vi "_f_IEEE754formatReverse.vi"(8 "error in (no error)":errorcluster, 9 "Number":sgl=-101.101 format="%.2f") -> (0 "error out":errorcluster, 1 "String":string="459CFFAE")   [LabVIEW 2013]
doc: "This VI shows how LabVIEW stores SGL floating-point numbers in memory in binary format. The 32-bit binary number is based on the following IEEE 754 format:\n\n1 bit for the SIGN\n8 bits for the EXPONENT\n23 bits for the MANTISSA\n\nThe formula for the conversion is the following:\n\nSGL = (-1)^SIGN * 1.MANTISSA * 2^(EXPONENT-127)\n\nYou can use this VI to convert SGL numbers to their binary storage equivalent, and vice versa."
panel:
  # "SGL to Binary Storage Format"
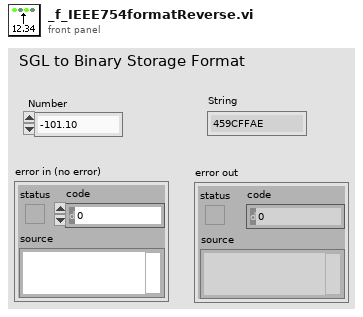
[diagram p1: front panel]
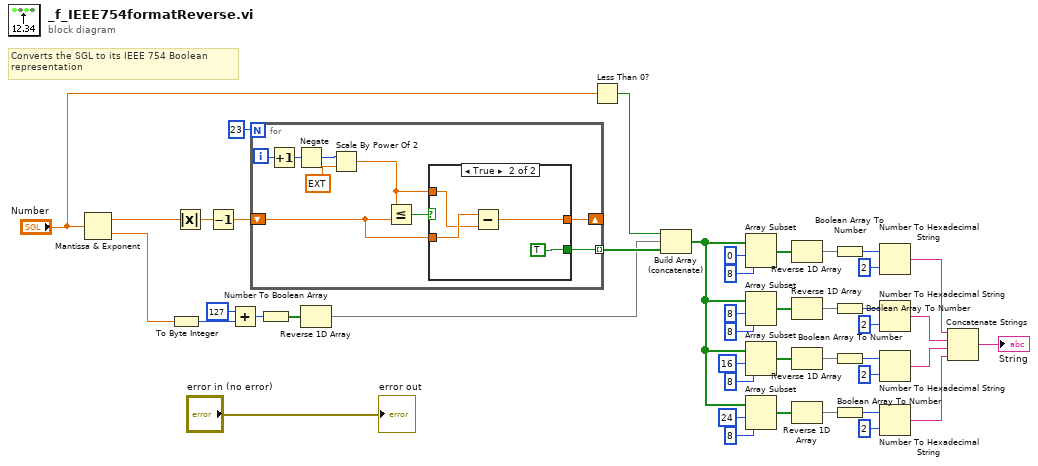
[diagram p0: block diagram]
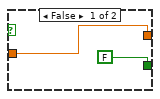
[diagram p2: hidden frame]
diagram:
  # "Converts the SGL to its IEEE 754 Boolean \nrepresentation"
  n1 = Mantissa & Exponent(0:"Number") -> (1:w35:sgl, 2:w38:sgl)
  n2 = To Byte Integer(number=w38) -> (8bit integer=w44:i8)
  n3 = Absolute Value(x=w35) -> (abs(x)=w36:sgl)
  n4 = Decrement(x=w36) -> (x-1=w40:sgl)
  n5 = Add(x=i8 127, y=w44) -> (x+y=w43:i8)
  n6 = for {
    N: 23 -> [_]
    shift-right: [w46] -> _
    shift-left: w40 -> [w48]
    tunnel: [w45] -> w33 mode=indexing
    i -> [w53]
    n7 = Increment(x=w53) -> (x+1=w52:i32)
    n8 = Negate(x=w52) -> (-x=w51:i32)
    n9 = Scale By Power Of 2(n=w51, x=ext 1.0) -> (x*2^n=w47:ext)
    n10 = Less Or Equal?(x=w47, y=w48) -> (x <= y?=w49:bool)
    n11 = case shown="True" w49 {
      tunnel: w48 -> [w54 w59]
      tunnel: w47 -> [_ w56]
      tunnel: [w54 w58] -> w46
      tunnel: [FALSE TRUE] -> w45
      frame False {
      }
      frame True {
        n12 = Subtract(x=w59, y=w56) -> (x-y=w58:ext)
      }
    }
  }
  n13 = Number To Boolean Array(number=w43) -> (Boolean array=w42:bool[])
  n14 = Reverse 1D Array(array=w42) -> (reversed array=w32:bool[])
  n15 = Less Than 0?(x="Number") -> (x < 0?=w34:bool)
  n16 = Build Array (concatenate)(w34, w32, w33) -> (w5:bool[])
  n17 = Array Subset(array=w5, index=0, length=8) -> (w22:bool[])
  n18 = Array Subset(array=w5, index=8, length=8) -> (w17:bool[])
  n19 = Array Subset(array=w5, index=16, length=8) -> (w15:bool[])
  n20 = Array Subset(array=w5, index=24, length=8) -> (w13:bool[])
  n21 = Reverse 1D Array(array=w22) -> (reversed array=w4:bool[])
  n22 = Reverse 1D Array(array=w17) -> (reversed array=w3:bool[])
  n23 = Reverse 1D Array(array=w15) -> (reversed array=w2:bool[])
  n24 = Reverse 1D Array(array=w13) -> (reversed array=w1:bool[])
  n25 = Boolean Array To Number(Boolean array=w4) -> (number=w21:u32)
  n26 = Boolean Array To Number(Boolean array=w3) -> (number=w18:u32)
  n27 = Boolean Array To Number(Boolean array=w2) -> (number=w16:u32)
  n28 = Boolean Array To Number(Boolean array=w1) -> (number=w14:u32)
  n29 = Number To Hexadecimal String(1:i16 2 ("width (-)"), 2:w21) -> (0:w20:string)
  n30 = Number To Hexadecimal String(1:i16 2 ("width (-)"), 2:w18) -> (0:w12:string)
  n31 = Number To Hexadecimal String(1:i16 2 ("width (-)"), 2:w16) -> (0:w11:string)
  n32 = Number To Hexadecimal String(1:i16 2 ("width (-)"), 2:w14) -> (0:w10:string)
  n33 = Concatenate Strings(w20, w12, w11, w10) -> (→"String":string)
  "error out" <- "error in (no error)"
